vi "Read Measured Voltage.vi"(8 "error in (no error)":errorcluster, 11 "VISA session":refnum<visa-resource-name>) -> (0 "error out":errorcluster, 2 "Voltage":dbl, 3 "dup VISA session":refnum<visa-resource-name>)   [LabVIEW 2011, in "Magna PSU.lvlib"]
uses:
  Magna PSU.lvlib
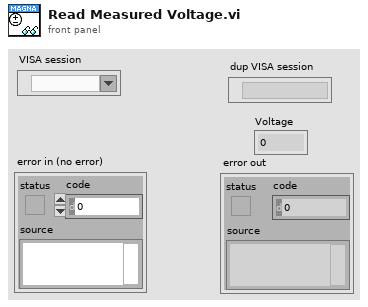
[diagram p1: front panel]
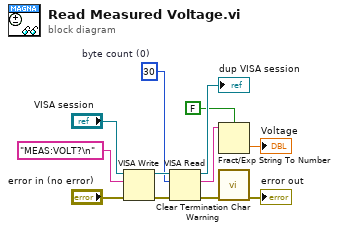
[diagram p0: block diagram]
diagram:
  w9 = u32 30  # byte count (0)
  n1 = VISA Write(VISA resource name="VISA session", write buffer="MEAS:VOLT?\n", error in (no error)="error in (no error)") -> (VISA resource name out=w11:refnum<visa-resource-name>, error out=w10:errorcluster)  [unwired: 1 out]
  n2 = VISA Read(VISA resource name=w11, byte count=w9, error in (no error)=w10) -> (VISA resource name out=→"dup VISA session":refnum<visa-resource-name>, read buffer=w2:string, error out=w5:errorcluster)  [unwired: 1 out]
  n3 = Fract/Exp String To Number(use system decimal point (T)=FALSE, string=w2) -> (number=→"Voltage":dbl)  [unwired: 2 in, 1 out]
  n4 = call "Clear Termination Char Warning.vi"("error in (no error)"=w5) -> ("error out"=→"error out":errorcluster)  [unwired: 10 in]
